vi "Process.vi"(8 "error in (no error)":errorcluster, 10 "Json Data":string, 11 "InferenceTCP in":refnum<class "InferenceTCP.lvclass">) -> (0 "error out":errorcluster, 3 "InferenceTCP out":refnum<class "InferenceTCP.lvclass">)   [LabVIEW 2021, in "InferenceTCP.lvlib" / "InferenceTCP.lvclass"]
uses:
  InferenceTCP.lvclass
  C:/Repos/Demo/Actors/AI Inference/Inference/Inference/Inference.lvclass
  InferenceTCP.lvclass/InferenceTCP.ctl
  Models/InferenceResultsModel.ctl
  Models/InferenceDataModel.ctl
  ad5c68d7-18df-410d-b4be-b7500ce97eba.vi
  122c796f-acd6-42ff-a738-eb890f4a0c5e.vi
  <vilib>/JDP Science/JSONtext/JSON text to Variant.vi
  <vilib>/JDP Science/JSONtext/Variant to JSON Text.vi
  <vilib>/JDP Science/JSONtext/LVClass Serializer/JSONtext LVClass Serializer.lvclass
  Inference/Inference/Inference.lvclass
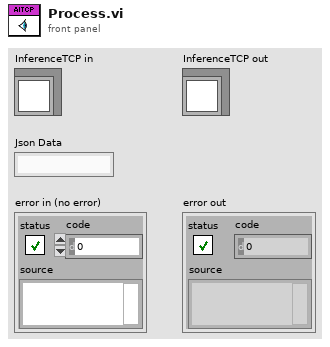
[diagram p1: front panel]
types:
  T1 = typedef "InferenceDataModel.ctl" = cluster{"guid":string, "images":string[]}
  T2 = typedef "InferenceResultsModel.ctl" = cluster{"guid":string, "results":cluster{"pass":bool, "class":string}[], "time":dbl}
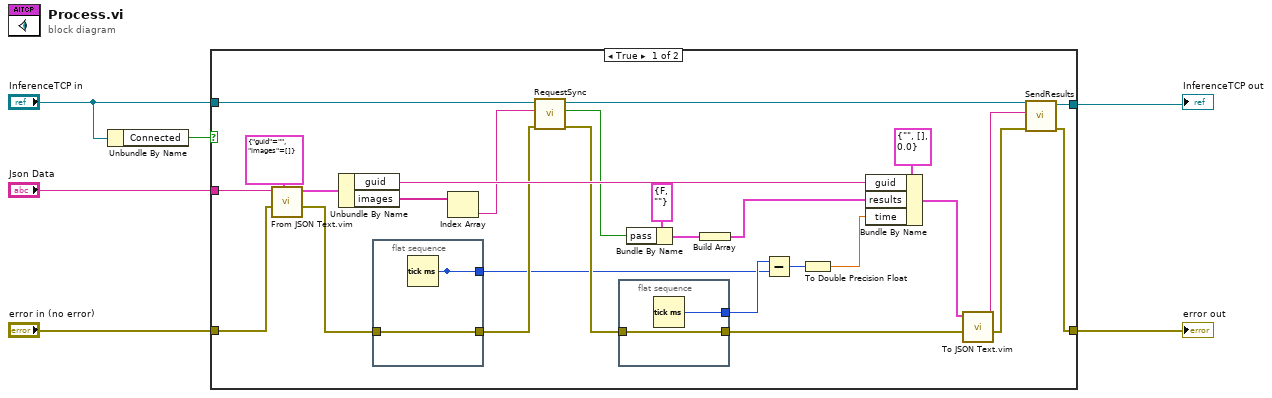
[diagram p0: block diagram]
diagram:
  n1 = Unbundle By Name("InferenceTCP in") -> ("Connected"=w3:bool)
  n2 = case shown="True" w3 {
    tunnel: "Json Data" -> [w33 _]
    tunnel: "error in (no error)" -> [w32 w38]
    tunnel: "InferenceTCP in" -> [w23 w39]
    tunnel: [w8 w39] -> w2
    tunnel: [w7 w38] -> w1
    frame True {
      n3 = call "From JSON Text.vim"("Data Type and Default Value"=T1 {"guid"="", "images"=[]} ("Data"), "error in (no error)"=w32, "JSON"=w33) -> ("error out"=w19:errorcluster, "Data out"=w30:T1)  [unwired: 7 in]
      n4 = Unbundle By Name(w30) -> ("guid"=w28:string, "images"=w22:string[])
      n5 = flat-sequence {
        tunnel: w19 -> [w37]
        tunnel: [w37] -> w18
        tunnel: [w36] -> _
        tunnel: [w36] -> w15
        frame #0 {
          n6 = Tick Count (ms)() -> (millisecond timer value=w36:u32)
        }
      }
      n7 = Index Array(array=w22) -> (element=w21:string)  [unwired: 1 in]
      n8 = call "RequestSync.vi"("error in (no error)"=w18, "Image Data"=w21, "InferenceTCP in"=w23) -> ("error out"=w17:errorcluster, "Result"=w20:bool, "InferenceTCP out"=w9:refnum<class "InferenceTCP.lvclass">)  [unwired: 6 in]
      n9 = flat-sequence {
        tunnel: w17 -> [w35]
        tunnel: [w35] -> w12
        tunnel: [w34] -> w16
        frame #0 {
          n10 = Tick Count (ms)() -> (millisecond timer value=w34:u32)
        }
      }
      n11 = Bundle By Name(cluster=cluster{"pass":bool, "class":string} {"pass"=FALSE, "class"=""} ("results"), "pass"=w20) -> (w26:cluster{"pass":bool, "class":string})
      n12 = Build Array(w26) -> (w25:cluster{"pass":bool, "class":string}[])
      n13 = Subtract(x=w16, y=w15) -> (x-y=w14:u32)
      n14 = To Double Precision Float(number=w14) -> (double precision float=w13:dbl)
      n15 = Bundle By Name(cluster=T2 {"guid"="", "results"=[], "time"=0.0} ("data"), "guid"=w28, "results"=w25, "time"=w13) -> (w24:T2)
      n16 = call "To JSON Text.vim"("error in (no error)"=w12, "Anything"=w24) -> ("error out"=w11:errorcluster, "<JSON>"=w10:string)  [unwired: 8 in]
      n17 = call "SendResults.vi"("error in (no error)"=w11, "Result Json"=w10, "Inference in"=w9) -> ("error out"=w7:errorcluster, "Inference out"=w8:refnum<class "InferenceTCP.lvclass">)  [unwired: 7 in]
    }
    frame False {
    }
  }
  "error out" <- w1
  "InferenceTCP out" <- w2
